vi "Set_Global_Settings.vi"(8 "error in (no error)":errorcluster, 10 "FIFO_PKT_SIZE":u16, 11 "VISA Refnum in":refnum<visa-resource-name>) -> (0 "error out":errorcluster, 3 "VISA Refnum out":refnum<visa-resource-name>)   [LabVIEW 2019]
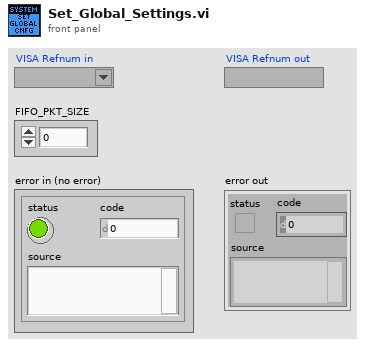
[diagram p1: front panel]
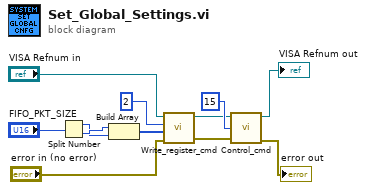
[diagram p0: block diagram]
diagram:
  n1 = Split Number(x="FIFO_PKT_SIZE") -> (hi(x)=w3:u8, lo(x)=w4:u8)
  n2 = Build Array(w4, w3) -> (w5:u8[])
  n3 = call "Write_register_cmd.vi"("Arty-7 Error In"="error in (no error)", "Data Array"=w5, "WrReg Addr"=u8 2, "Arty-7 VISA In"="VISA Refnum in") -> ("Arty-7 Error out"=w7:errorcluster, "Arty-7 VISA out"=w6:refnum<visa-resource-name>)  [unwired: 4 in, 2 out]
  n4 = call "Control_cmd.vi"("Arty-7 Error In"=w7, "Control Command"=u8 15, "Arty-7 VISA In"=w6) -> ("Arty-7 Error out"=→"error out":errorcluster, "Arty-7 VISA out"=→"VISA Refnum out":refnum<visa-resource-name>)  [unwired: 2 in, 2 out]
